vi "Get Controller Information.vi"(4 "Expose System Hardware Reference":bool caption="Expose System Hardware Reference (F)", 6 "Network Adapters":bool caption="Network Adapters (F)", 8 "error in":errorcluster, 11 "Session in":refnum<k21>="localhost") -> (0 "error out":errorcluster, 2 "Network Device":T1={"System Hardware Reference"=refnum, "Device Information"={"Resource"="", "Vendor Name"="", "Product Name"="", "Product ID"=0, "Serial Number"="", "Device Class"="", "System Start Time"=timestamp(0 s since 1904-01-01), "Current Time"=timestamp(0 s since 1904-01-01), "Time Zone"="", "Firmware Revision"="", "Image Title"="", "Image Version"="", "System Status"="", "Credential type"=enum."None/Unlocked", "User Added"=FALSE}, "Primary Network Adapter"={"IP Address"="", "MAC Address"="", "IP Address Request Mode"=1, "SubnetMask"="", "Gateway"="", "DNS Server"="", "Adapter Mode"=1, "Adapter Type"=1}, "Secondary Network Adapters"=[]} {"Primary Network Adapter"."IP Address Request Mode" items=["Static"=1, "DHCP/Link Local"=2, "Link-Local Only"=4, "DHCP Only"=8]; "Primary Network Adapter"."Adapter Type" items=["Ethernet"=1, "WLAN"=2]; "Primary Network Adapter"."Adapter Mode" items=["Disabled"=1, "TCP/IP Ethernet"=2, "Deterministic"=4, "EtherCAT"=8, "TCP/IP WLAN Connect"=32, "TCP/IP WLAN Create"=64]; "Secondary Network Adapters"."IP Address Request Mode" items=["Static"=1, "DHCP/Link Local"=2, "Link-Local Only"=4, "DHCP Only"=8]; "Secondary Network Adapters"."Adapter Type" items=["Disabled"=1, "TCP/IP Ethernet"=2, "Deterministic"=4, "EtherCAT"=8, "TCP/IP WLAN Connect"=32, "TCP/IP WLAN Create"=64]; "Secondary Network Adapters"."Adapter Mode" items=["Disabled"=1, "TCP/IP Ethernet"=2, "Deterministic"=4, "EtherCAT"=8, "TCP/IP WLAN Connect"=32, "TCP/IP WLAN Create"=64]; "Device Information"."Product ID" format="%.0x"}, 3 "Session out":refnum<k21>="localhost")   [LabVIEW 2015, in "SMI.lvlib" / "Controller.lvclass"]
uses:
  Controller.lvclass
  Distributed Devices/Controls/NetworkDevice.ctl
  Distributed Devices/Controls/DeviceInformation.ctl
  Distributed Devices/Controls/NetworkAdapterSettings.ctl
  <vilib>/nisyscfg/Find Hardware.vi
  <vilib>/nisyscfg/Close (Resources).vi
  <vilib>/nisyscfg/Close (Filter).vi
  <vilib>/nisyscfg/nisyscfg.lvlib
  <resource>/objmgr/niflexriosae.rc
  Distributed Devices/Device.lvclass
  <resource>/objmgr/nisysapi.rc
  RT Management.lvlib
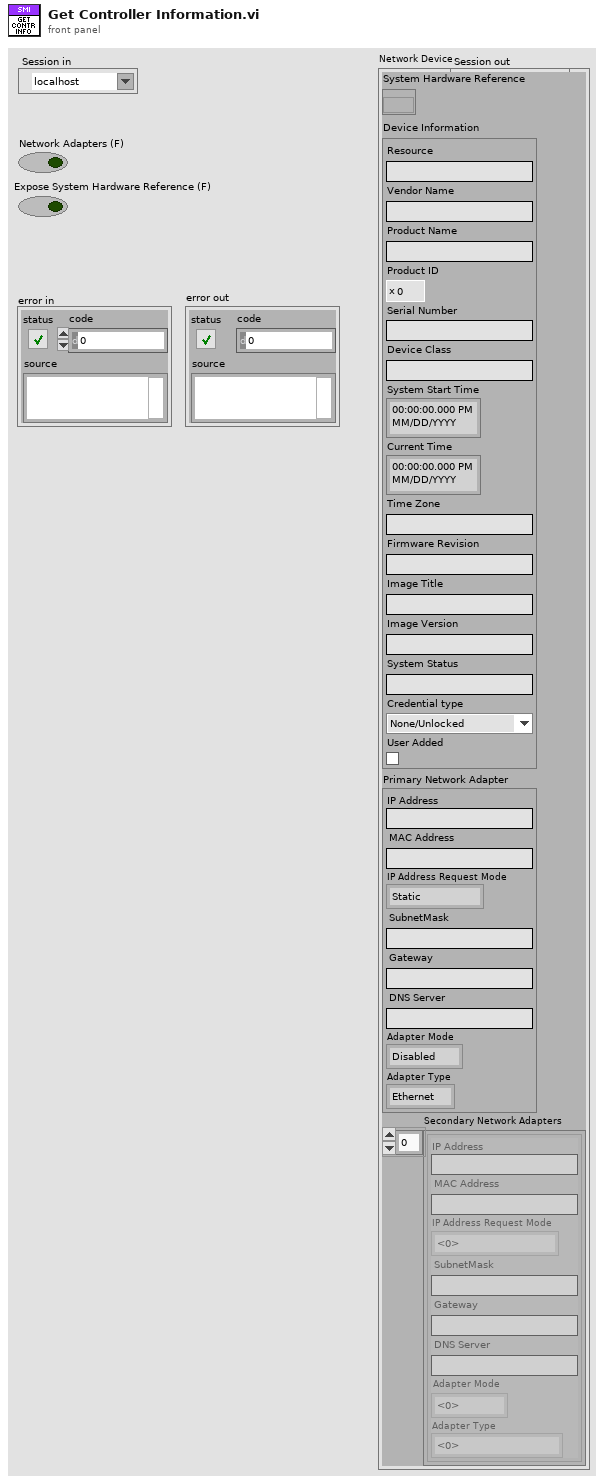
[diagram p1: front panel]
types:
  T1 = typedef "SMI.lvlib/Device.lvclass/NetworkDevice.ctl" = cluster{"System Hardware Reference":refnum<k20>, "Device Information":T2, "Primary Network Adapter":T3, "Secondary Network Adapters":T3[]}
  T2 = typedef "SMI.lvlib/Device.lvclass/DeviceInformation.ctl" = cluster{"Resource":string, "Vendor Name":string, "Product Name":string, "Product ID":u32, "Serial Number":string, "Device Class":string, "System Start Time":timestamp, "Current Time":timestamp, "Time Zone":string, "Firmware Revision":string, "Image Title":string, "Image Version":string, "System Status":string, "Credential type":enum16{"None/Unlocked", "FTP Password", "NIAuth Credentials"}, "User Added":bool}
  T3 = typedef "SMI.lvlib/Device.lvclass/NetworkAdapterSettings.ctl" = cluster{"IP Address":string, "MAC Address":string, "IP Address Request Mode":u32, "SubnetMask":string, "Gateway":string, "DNS Server":string, "Adapter Mode":u32, "Adapter Type":u32}
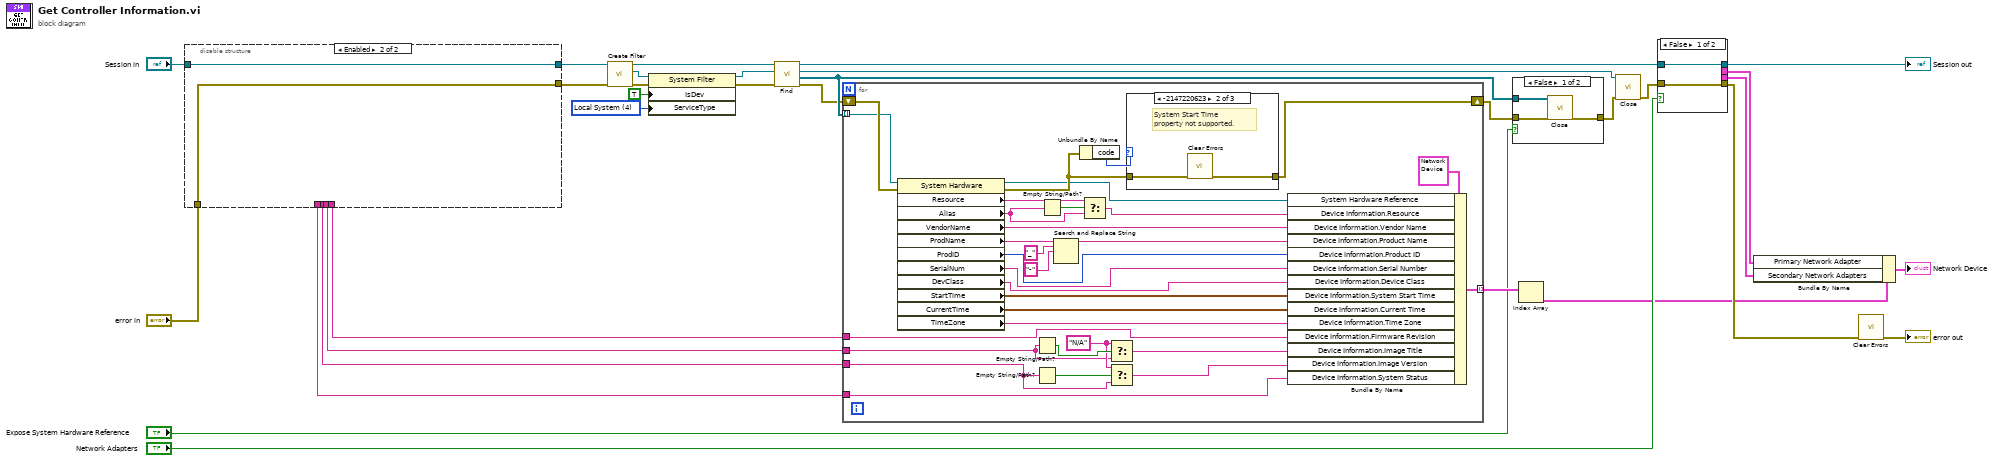
[diagram p0: block diagram]
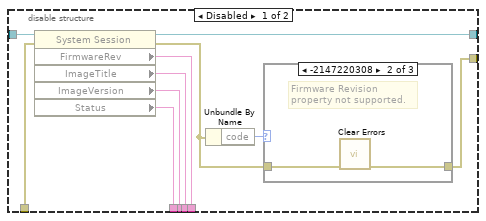
[diagram p2: hidden frame]
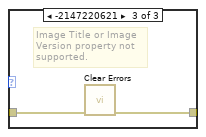
[diagram p4: hidden frame]
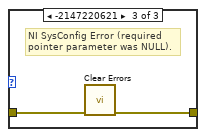
[diagram p7: hidden frame]
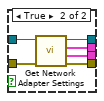
[diagram p8: hidden frame]
diagram:
  w2 = u32 4 items=["NI Network Resource", "NI Real-Time", "NI System Configuration", "NI Web Interface", "Local System", "Local Network Adapter", "Local Time Keeper", "Local Time Reference", "LXI Instrument", "Local FPGA"] ("Service Type")
  n1 = disable-structure shown="Enabled" {
    disable-tunnel: "error in" -> [w42 w48]
    disable-tunnel: "Session in" -> [w41 w49]
    disable-tunnel: [w40 _] -> w24
    disable-tunnel: [w39 _] -> w23
    disable-tunnel: [w38 _] -> w22
    disable-tunnel: [w35 _] -> w15
    disable-tunnel: [w34 w48] -> w7
    disable-tunnel: [w33 w49] -> w6
    frame Disabled {
      n2 = property class="System Session"(reference=w41, error in=w42) -> (reference out=w33:refnum<k21>, error out=w37:errorcluster, "FirmwareRev"=w35:string, "ImageTitle"=w38:string, "ImageVersion"=w40:string, "Status"=w39:string)
      n3 = Unbundle By Name(w37) -> ("code"=w36:i32)
      n4 = case shown="-2147220308" w36 {
        tunnel: w37 -> [w43 w45 w47]
        tunnel: [w43 w44 w46] -> w34
        frame Default {
        }
        frame -2147220308 {
          # "Firmware Revision\nproperty not supported."
          n5 = call <vilib>:"Clear Errors.vi"("error in (no error)"=w45) -> ("error out"=w44:errorcluster)  [unwired: 5 in, 1 out]
        }
        frame -2147220621 {
          # "Image Title or Image\nVersion property not \nsupported."
          n6 = call <vilib>:"Clear Errors.vi"("error in (no error)"=w47) -> ("error out"=w46:errorcluster)  [unwired: 5 in, 1 out]
        }
      }
    }
    frame Enabled {
    }
  }
  n7 = call <vilib>:"Create Filter.vi"("error in (no error)"=w7, "Session in"=w6) -> ("error out"=w10:errorcluster, "Filter out"=w9:refnum<k20>, "Session out"=w5:refnum<k21>)  [unwired: 7 in]
  n8 = property class="System Filter"(reference=w9, error in=w10, "IsDev"=TRUE ("Is Device"), "ServiceType"=w2) -> (reference out=w4:refnum<k20>, error out=w8:errorcluster)
  n9 = call-poly <vilib>:"Find.vi"("error in (no error)"=w8, "Filter in"=w4, "Session in"=w5) -> ("error out"=w14:errorcluster, "Resources out"=w18:refnum<k20>[], "Filter out"=w19:refnum<k20>, "Session out"=w26:refnum<k21>)  [unwired: 5 in]
  n10 = for {
    tunnel: w24 -> [w53]
    tunnel: w23 -> [w81]
    tunnel: w22 -> [w52]
    tunnel: w18 -> [w58] mode=indexing
    tunnel: [w76] -> w12 mode=indexing
    tunnel: w15 -> [w75]
    shift-right: [w78] -> w17
    shift-left: w14 -> [w74]
    w54 = "N/A"
    n11 = property class="System Hardware"(reference=w58, error in=w74) -> (reference out=w57:refnum<k20>, error out=w80:errorcluster, "Resource"=w71:string, "Alias"=w70:string, "VendorName"=w67:string, "ProdName"=w65:string, "ProdID"=w62:u32, "SerialNum"=w63:string, "DevClass"=w59:string, "StartTime"=w68:timestamp, "CurrentTime"=w72:timestamp, "TimeZone"=w73:string)
    n12 = Empty String/Path?(string/path=w52) -> (empty?=w55:bool)
    n13 = Empty String/Path?(string/path=w53) -> (empty?=w56:bool)
    n14 = Empty String/Path?(string/path=w70) -> (empty?=w69:bool)
    n15 = Search and Replace String(input string=w65, search string="_", replace string="-" ("replace string (\"\")")) -> (result string=w64:string)  [unwired: 5 in, 3 out]
    n16 = Unbundle By Name(w80) -> ("code"=w79:i32)
    n17 = Select(t=w71, s=w69, f=w70) -> (s? t:f=w66:string)
    n18 = Select(t=w54, s=w55, f=w52) -> (s? t:f=w50:string)
    n19 = Select(t=w54, s=w56, f=w53) -> (s? t:f=w51:string)
    n20 = case shown="-2147220623" w79 {
      tunnel: w80 -> [w82 w84 w86]
      tunnel: [w82 w83 w85] -> w78
      frame Default {
      }
      frame -2147220623 {
        # "System Start Time\nproperty not supported."
        n21 = call <vilib>:"Clear Errors.vi"("error in (no error)"=w84) -> ("error out"=w83:errorcluster)  [unwired: 5 in, 1 out]
      }
      frame -2147220621 {
        # "NI SysConfig Error (required\npointer parameter was NULL)."
        n22 = call <vilib>:"Clear Errors.vi"("error in (no error)"=w86) -> ("error out"=w85:errorcluster)  [unwired: 5 in, 1 out]
      }
    }
    n23 = Bundle By Name(cluster=T1 {"System Hardware Reference"=refnum, "Device Information"={"Resource"="", "Vendor Name"="", "Product Name"="", "Product ID"=0, "Serial Number"="", "Device Class"="", "System Start Time"=timestamp(0 s since 1904-01-01), "Current Time"=timestamp(0 s since 1904-01-01), "Time Zone"="", "Firmware Revision"="", "Image Title"="", "Image Version"="", "System Status"="", "Credential type"=enum."None/Unlocked", "User Added"=FALSE}, "Primary Network Adapter"={"IP Address"="", "MAC Address"="", "IP Address Request Mode"=1, "SubnetMask"="", "Gateway"="", "DNS Server"="", "Adapter Mode"=1, "Adapter Type"=1}, "Secondary Network Adapters"=[]} ("Network Device"), "System Hardware Reference"=w57, "Device Information.Resource"=w66, "Device Information.Vendor Name"=w67, "Device Information.Product Name"=w64, "Device Information.Product ID"=w62, "Device Information.Serial Number"=w63, "Device Information.Device Class"=w59, "Device Information.System Start Time"=w68, "Device Information.Current Time"=w72, "Device Information.Time Zone"=w73, "Device Information.Firmware Revision"=w75, "Device Information.Image Title"=w50, "Device Information.Image Version"=w51, "Device Information.System Status"=w81) -> (w76:T1)
  }
  n24 = case shown="False" "Expose System Hardware Reference" {
    tunnel: [w89 w90] -> w20
    tunnel: w18 -> [w88 _]
    tunnel: w17 -> [w87 w90]
    frame False {
      n25 = call-poly <vilib>:"Close.vi"("error in (no error)"=w87, "Resources in"=w88) -> ("error out"=w89:errorcluster)  [unwired: 9 in]
    }
    frame True {
    }
  }
  n26 = Index Array(array=w12) -> (element=w13:T1)  [unwired: 1 in]
  n27 = call-poly <vilib>:"Close.vi"("error in (no error)"=w20, "Filter in"=w19) -> ("error out"=w25:errorcluster)  [unwired: 9 in]
  n28 = case shown="False" "Network Adapters" {
    tunnel: w26 -> [w92 w98]
    tunnel: w25 -> [w91 w97]
    tunnel: [_ w96] -> w21
    tunnel: [w92 w95] -> w30
    tunnel: [w91 w94] -> w16
    tunnel: [_ w93] -> w1
    frame False {
    }
    frame True {
      n29 = call "Get Network Adapter Settings.vi"("error in"=w97, "Refnum in"=w98) -> ("error out"=w94:errorcluster, "Secondary Network Adapters"=w93:T3[], "Primary Network Adapter"=w96:T3, "Refnum out"=w95:refnum<k21>)  [unwired: 6 in]
    }
  }
  "Session out" <- w30
  n30 = Bundle By Name(cluster=w13, "Primary Network Adapter"=w21, "Secondary Network Adapters"=w1) -> (→"Network Device":T1)
  n31 = call <vilib>:"Clear Errors.vi"("error in (no error)"=w16) -> ("error out"=→"error out":errorcluster)  [unwired: 5 in, 1 out]
